vi "Play Error Sound.vi"(15 "Error In":errorcluster) -> (14 "Error Out":errorcluster)   [LabVIEW 2021, in "Sound.lvlib"]
uses:
  System Sounds List.ctl
  Sound.lvlib
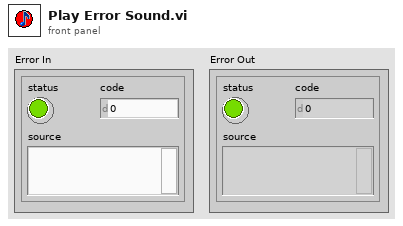
[diagram p1: front panel]
types:
  T1 = typedef "Sound.lvlib/System Sounds List.ctl" = enum16{"Alarm01", "Alarm02", "Alarm03", "Alarm04", "Alarm05", "Alarm06", "Alarm07", "Alarm08", "Alarm09", "Alarm10", "chimes", "chord", "ding", "notify", "recycle", "Ring01", "Ring02", "Ring03", "Ring04", "Ring05", "Ring06", "Ring07", "Ring08", "Ring09", "Ring10", "ringout", "Speech Off", "Speech On", "Speech Sleep", "tada", "Windows Background", "Windows Balloon", "Windows Battery Critical", "Windows Battery Low", "Windows Critical Stop", "Windows Default", "Windows Ding", "Windows Error", "Windows Exclamation", "Windows Feed Discovered", "Windows Foreground", "Windows Hardware Fail", "Windows Hardware Insert", "Windows Hardware Remove", "Windows Information Bar", "Windows Logoff Sound", "Windows Logon", "Windows Menu Command", "Windows Message Nudge", "Windows Minimize", "Windows Navigation Start", "Windows Notify Calendar", "Windows Notify Email", "Windows Notify Messaging", "Windows Notify System Generic", "Windows Notify", "Windows Pop-up Blocked", "Windows Print complete", "Windows Proximity Connection", "Windows Proximity Notification", "Windows Recycle", "Windows Restore", "Windows Ringin", "Windows Ringout", "Windows Shutdown", "Windows Startup", "Windows Unlock", "Windows User Account Control"}
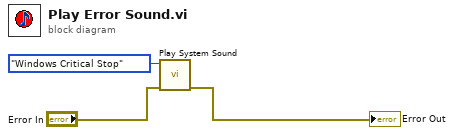
[diagram p0: block diagram]
diagram:
  n1 = call "Play System Sound.vi"("Error In"="Error In", "Windows Sound"=System_Sounds_List."Windows Critical Stop") -> ("Error Out"=→"Error Out":errorcluster)  [unwired: 9 in]
